vi "randomInRange.vi"(10 "numMin":dbl=100.0, 11 "numMax":dbl) -> (3 "RandomNumber":dbl)   [LabVIEW 2014]
panel:
  out "Waveform Chart":dbl(graph)
  in  "stop":bool
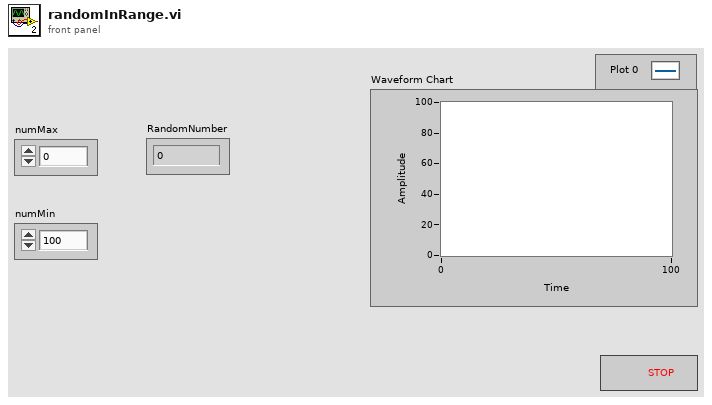
[diagram p1: front panel]
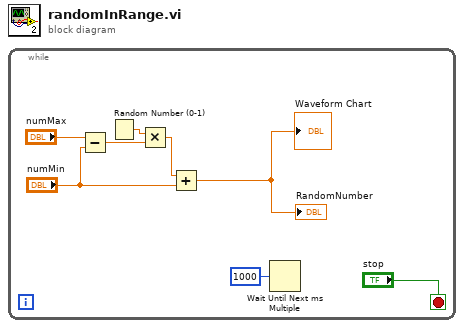
[diagram p0: block diagram]
diagram:
  n1 = while {
    stop <- "stop" stop-if-true
    n2 = Subtract(x="numMax", y="numMin") -> (x-y=w6:dbl)
    n3 = Random Number (0-1)() -> (number: 0 to 1=w7:dbl)
    n4 = Multiply(x=w7, y=w6) -> (x*y=w4:dbl)
    n5 = Add(x=w4, y="numMin") -> (x+y=→"RandomNumber" →"Waveform Chart":dbl)
    n6 = Wait Until Next ms Multiple(millisecond multiple=u32 1000) -> ()  [unwired: 1 out]
  }
